vi "test_queue.vi"() -> ()   [LabVIEW 2012]
doc: "Use this template to build a producer/consumer design pattern. Use this template when you need to execute a process, such as data analysis, when a data source, such as a triggered acquisition, produces data at an uneven rate and you need to execute the process when the data becomes available."
panel:
  in  "stop restore":bool
  in  "stop save":bool
  out "Waveform Chart 2":dbl(graph)
  out "Waveform Chart":dbl(graph)
  in  "stop":bool
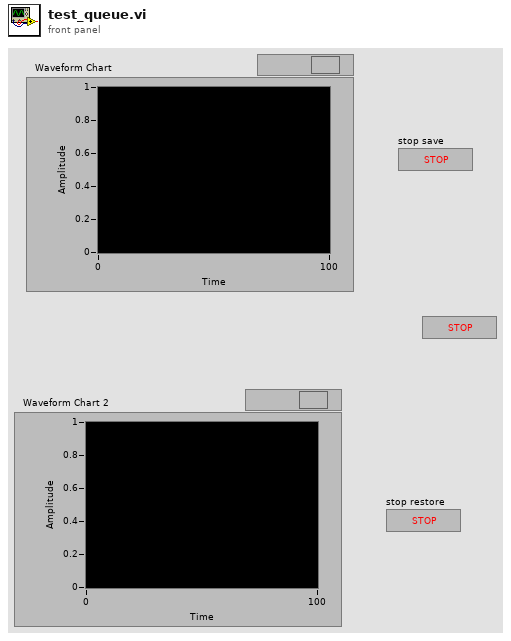
[diagram p1: front panel]
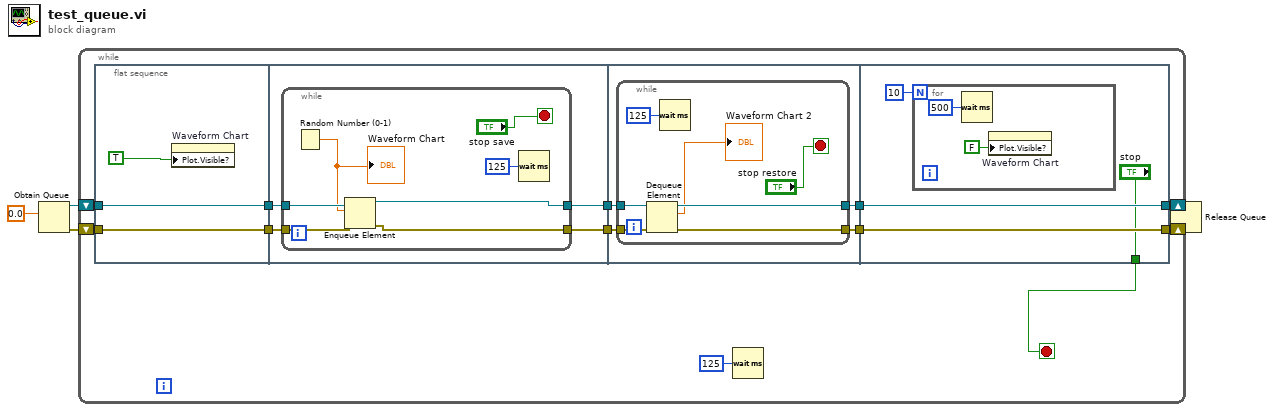
[diagram p0: block diagram]
diagram:
  n1 = Obtain Queue(element data type=0.0) -> (queue out=w5:refnum<queue>, error out=w4:errorcluster)  [unwired: 4 in, 1 out]
  n2 = while {
    shift-right: [w14] -> w2
    shift-left: w4 -> [w16]
    shift-right: [w15] -> w3
    shift-left: w5 -> [w17]
    stop <- w8 stop-if-true
    n3 = flat-sequence {
      tunnel: w16 -> [w19]
      tunnel: w17 -> [w20]
      tunnel: [w20] -> w7
      tunnel: [w19] -> w6
      tunnel: [w22] -> w13
      tunnel: [w21] -> w12
      tunnel: w7 -> [w24]
      tunnel: w6 -> [w23]
      tunnel: w13 -> [w35]
      tunnel: w12 -> [w33]
      tunnel: [w34] -> w10
      tunnel: [w32] -> w9
      tunnel: [w45] -> w14
      tunnel: [w46] -> w15
      tunnel: w10 -> [w46]
      tunnel: w9 -> [w45]
      tunnel: ["stop"] -> w8
      frame #0 {
        n4 = property on="Waveform Chart" class="WFChart (strict)"("Plot.Visible?"=TRUE ("Plot.Visible")) -> ()  [unwired: 2 in, 2 out]
      }
      frame #1 {
        n5 = while {
          tunnel: w24 -> [w31]
          tunnel: w23 -> [w30]
          tunnel: [w29] -> w22
          tunnel: [w27] -> w21
          stop <- "stop save" stop-if-true
          n6 = Random Number (0-1)() -> (number: 0 to 1=w28:dbl)
          "Waveform Chart" <- w28
          n7 = Enqueue Element(queue=w31, element=w28, error in (no error)=w30) -> (queue out=w29:refnum<queue>, error out=w27:errorcluster)  [unwired: 1 in, 1 out]
          n8 = Wait (ms)(milliseconds to wait=u32 125) -> ()  [unwired: 1 out]
        }
      }
      frame #2 {
        n9 = while {
          tunnel: w35 -> [w42]
          tunnel: [w41] -> w34
          tunnel: w33 -> [w40]
          tunnel: [w39] -> w32
          stop <- "stop restore" stop-if-true
          n10 = Dequeue Element(queue=w42, error in (no error)=w40) -> (queue out=w41:refnum<queue>, element=→"Waveform Chart 2":dbl, error out=w39:errorcluster)  [unwired: 1 in, 1 out]
          n11 = Wait (ms)(milliseconds to wait=u32 125) -> ()  [unwired: 1 out]
        }
      }
      frame #3 {
        n12 = for {
          N: 10 -> [_]
          n13 = Wait (ms)(milliseconds to wait=u32 500) -> ()  [unwired: 1 out]
          n14 = property on="Waveform Chart" class="WFChart (strict)"("Plot.Visible?"=FALSE ("Plot.Visible")) -> ()  [unwired: 2 in, 2 out]
        }
      }
    }
    n15 = Wait (ms)(milliseconds to wait=u32 125) -> ()  [unwired: 1 out]
  }
  n16 = Release Queue(queue=w3, error in (no error)=w2) -> ()  [unwired: 1 in, 3 out]
